vi "Create Tree Priv.vi"(8 "Error In":errorcluster, 9 "Name":string, 11 "Tree Dictionary In":variant) -> (0 "Error Out":errorcluster, 2 "Unique ID":string, 3 "Tree Dictionary Out":variant)   [LabVIEW 2020, in "NI_VIAnCFGDataStructure.lvlib" / "Tree.lvclass"]
uses:
  <vilib>/addons/analyzer/VIAnCFGDataStructure/Tree Manager/Tree.lvclass
  <vilib>/addons/analyzer/VIAnCFGDataStructure/Tree Manager/Typedefs/Tree Cluster.ctl
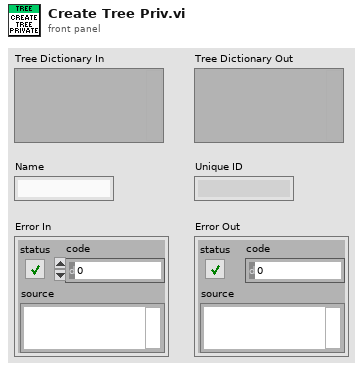
[diagram p1: front panel]
types:
  T1 = typedef "NI_VIAnCFGDataStructure.lvlib/Tree.lvclass/Tree Cluster.ctl" = cluster{"Unique ID":string, "Parent ID":string, "Child IDs":string[], "Name":string, "MetaData":string, "Data IDs":string[]}
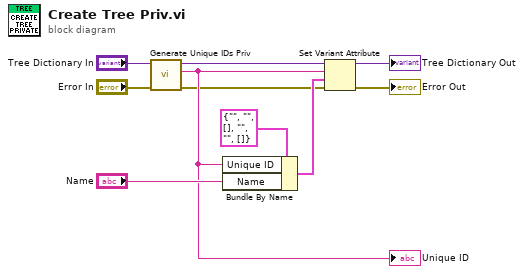
[diagram p0: block diagram]
diagram:
  n1 = call <vilib>:"Generate Unique IDs Priv.vi"("Error In"="Error In", "Tree Dictionary"="Tree Dictionary In") -> ("Error Out"=w5:errorcluster, "First ID"=w9:string, "Tree Dictionary Out"=w8:variant)  [unwired: 6 in, 1 out]
  "Unique ID" <- w9
  n2 = Bundle By Name(cluster=T1 {"Unique ID"="", "Parent ID"="", "Child IDs"=[], "Name"="", "MetaData"="", "Data IDs"=[]} ("Cluster of class private data"), "Unique ID"=w9, "Name"="Name") -> (w7:T1)
  n3 = Set Variant Attribute(Variant=w8, name=w9, value=w7, error in=w5) -> (Variant out=→"Tree Dictionary Out":variant, error out=→"Error Out":errorcluster)  [unwired: 1 out]
